vi "OAT Polar Transfer Cursor Position to EU.vi"(7 "polar settings":T1={"polar attributes"={"maximum"=2.0, "minimum"=0.0, "clip to min"=FALSE, "log"=FALSE, "grid color"=3381657, "plot color"=16711680, "fmt and prec"={"format"=enum."Decimal", "precision"=2}, "visible section"=4}, "desired font(Application)"=enum."Application Font", "[user-specified font]"={"Font Name:"="", "Size"=0, "Strikeout?"=FALSE, "Italic?"=FALSE, "Underline?"=FALSE, "Outline?"=FALSE, "Shadow?"=FALSE, "Bold?"=FALSE}} {"polar attributes"."minimum" format="%.2f"; "polar attributes"."maximum" format="%.2f"}, 9 "picture \ndimensions (w,h)":cluster{"width":i16, "height":i16}, 10 "grid measurements":T2 {"end angle" format="%.2f"; "start angle" format="%.2f"; "scale factors"."b" format="%.2f"; "scale factors"."a" format="%.2f"}, 11 "XY Graph":refnum<vi>) -> (3 "Cursor List (EU position]":T3(array[cluster]) {"Location"."phase" format="%.2f"; "Location"."mag" format="%.2f"}, 5 "polar settings out":T1={"polar attributes"={"maximum"=2.0, "minimum"=0.0, "clip to min"=FALSE, "log"=FALSE, "grid color"=3381657, "plot color"=16711680, "fmt and prec"={"format"=enum."Decimal", "precision"=2}, "visible section"=4}, "desired font(Application)"=enum."Application Font", "[user-specified font]"={"Font Name:"="", "Size"=0, "Strikeout?"=FALSE, "Italic?"=FALSE, "Underline?"=FALSE, "Outline?"=FALSE, "Shadow?"=FALSE, "Bold?"=FALSE}} {"polar attributes"."minimum" format="%.2f"; "polar attributes"."maximum" format="%.2f"})   [LabVIEW 2017]
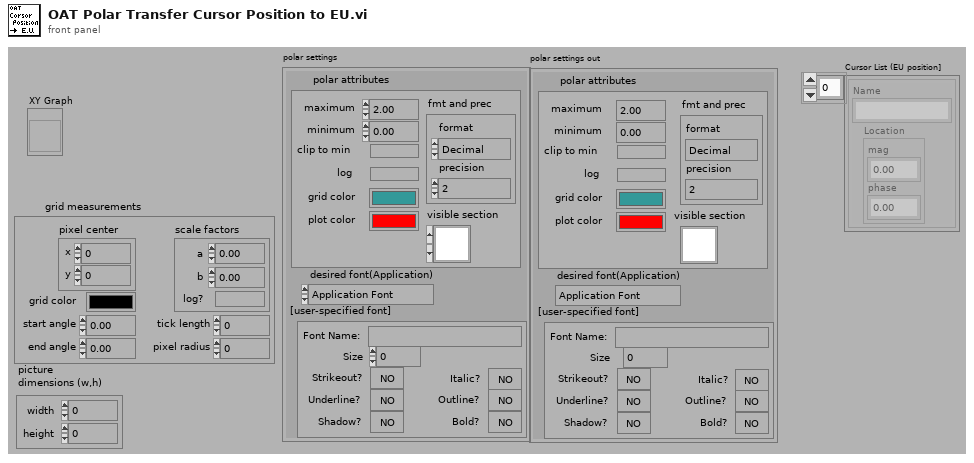
[diagram p1: front panel]
types:
  T1 = cluster{"polar attributes":cluster{"maximum":dbl, "minimum":dbl, "clip to min":bool, "log":bool, "grid color":u32, "plot color":u32, "fmt and prec":cluster{"format":enum8{"Decimal", "Scientific", "Engineering", "Binary", "Octal", "Hex"}, "precision":u8}, "visible section":u16}, "desired font(Application)":enum16{"User-specified Font", "Application Font", "System Font", "Dialog Font"}, "[user-specified font]":cluster{"Font Name:":string, "Size":i16, "Strikeout?":bool, "Italic?":bool, "Underline?":bool, "Outline?":bool, "Shadow?":bool, "Bold?":bool}}
  T2 = cluster{"pixel center":cluster{"x":i16, "y":i16}, "scale factors":cluster{"a":dbl, "b":dbl, "log?":bool}, "grid color":u32, "start angle":dbl, "end angle":dbl, "tick length":i16, "pixel radius":i32}
  T3 = cluster{"Name":string, "Location":cluster{"mag":dbl, "phase":dbl}}[]
  T4 = cluster{"Name":string, "Color":u32, "Style":u8, "Point Style":u8, "Name Visible":bool, "Allow Drag":bool, "Lock Style":u32, "Plot":u32, "Index":i32, "Position":cluster{"X":dbl, "Y":dbl}}[]
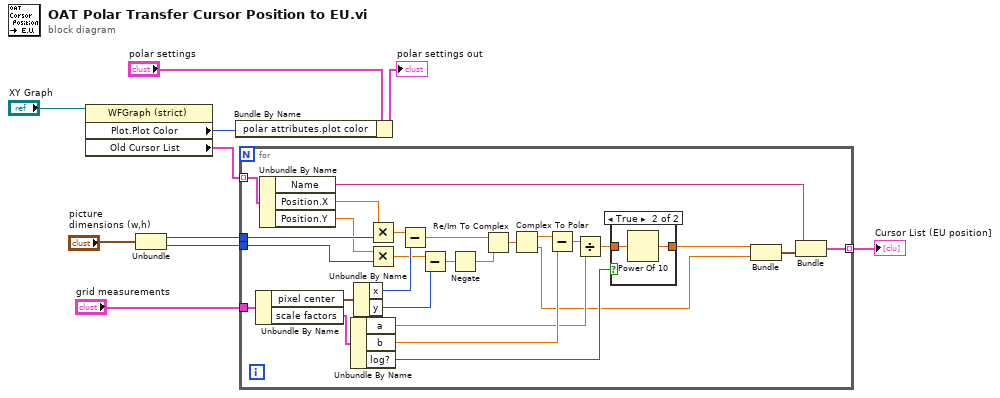
[diagram p0: block diagram]
diagram:
  n1 = property on="Property Node" class="WFGraph (strict)"(reference="XY Graph") -> ("Plot.Plot Color"=w9:u32, "Old Cursor List"=w7:T4)  [unwired: 1 in, 2 out]
  n2 = Unbundle("picture \ndimensions (w,h)") -> ("width"=w2:i16, "height"=w1:i16)
  n3 = Bundle By Name(cluster="polar settings", "polar attributes.plot color"=w9) -> (→"polar settings out":T1)
  n4 = for {
    tunnel: w7 -> [w16] mode=indexing
    tunnel: w2 -> [w36]
    tunnel: w1 -> [w34]
    tunnel: "grid measurements" -> [w32]
    tunnel: [w13] -> w5 mode=indexing
    n5 = Unbundle By Name(w32) -> ("pixel center"=w31:cluster{"x":i16, "y":i16}, "scale factors"=w22:cluster{"a":dbl, "b":dbl, "log?":bool})
    n6 = Unbundle By Name(w16) -> ("Name"=w14:string, "Position.X"=w37:dbl, "Position.Y"=w35:dbl)
    n7 = Unbundle By Name(w22) -> ("a"=w19:dbl, "b"=w21:dbl, "log?"=w18:bool)
    n8 = Unbundle By Name(w31) -> ("x"=w29:i16, "y"=w27:i16)
    n9 = Multiply(x=w37, y=w36) -> (x*y=w30:dbl)
    n10 = Multiply(x=w35, y=w34) -> (x*y=w28:dbl)
    n11 = Subtract(x=w30, y=w29) -> (x-y=w25:dbl)
    n12 = Subtract(x=w28, y=w27) -> (x-y=w26:dbl)
    n13 = Negate(x=w26) -> (-x=w24:dbl)
    n14 = Re/Im To Complex(1:w24, 2:w25) -> (0:w33:cdb)
    n15 = Complex To Polar(r * e^(i*theta)=w33) -> (r=w23:dbl, theta=w11:dbl)
    n16 = Subtract(x=w23, y=w21) -> (x-y=w20:dbl)
    n17 = Divide(x=w20, y=w19) -> (x/y=w17:dbl)
    n18 = case shown="True" w18 {
      tunnel: w17 -> [w38 w40]
      tunnel: [w38 w39] -> w12
      frame False {
      }
      frame True {
        n19 = Power Of 10(x=w40) -> (10^x=w39:dbl)
      }
    }
    n20 = Bundle(w12, w11) -> (w15:cluster{dbl, dbl})  [unwired: 1 in]
    n21 = Bundle("Name"=w14, w15) -> (w13:cluster{"Name":string, cluster{dbl, dbl}})  [unwired: 1 in]
  }
  "Cursor List (EU position]" <- w5
